vi "StartMeas.vi"(8 "error in (no error)":errorcluster, 11 "ChromaAcLoad in":refnum<class "ChromaAcLoad.lvclass">) -> (0 "error out":errorcluster, 3 "ChromaAcLoad out":refnum<class "ChromaAcLoad.lvclass">)   [LabVIEW 2018, in "AcPwrPlugins.lvlib" / "ChromaAcLoad.lvclass"]
uses:
  ChromaAcLoad.lvclass
  C:/Users/ico/Documents/Projects/NistPluggableModules/AcPwr/AcPwrPlugins/AcPwrBaseClass/AcPwrBase.lvclass
  AcPwrBaseClass/AcPwrBase.lvclass/AcPwrBase.ctl
  AcPwrBaseClass/Accessors/Read BaseMeasures.vi
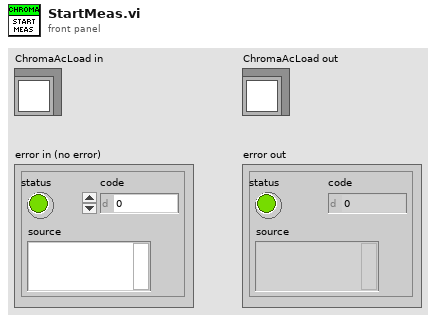
[diagram p1: front panel]
types:
  T1 = typedef "AcPwrPlugins.lvlib/AcPwrBase.lvclass/BaseMeasure.ctl" = cluster{"Handle":string, "Name":string, "Enabled":bool, "Result":dbl, "MeasType":T2, "btnMeasFetch":bool, "Hold Peak?":bool}
  T2 = typedef "AcPwrPlugins.lvlib/AcPwrBase.lvclass/MeasType.ctl" = enum16{"Voltage RMS L-N", "Current RMS", "Frequency", "Voltage DC", "Current DC", "Power Factor", "Current Peak", "Power VA", "Real Power", "Voltage THD", "Voltage EHD", "Voltage OHD", "Current THD", "Current EHD", "Current OHD", "Voltage RMS L-L", "Phase Angle", "Power DC", "Crest Factor"}
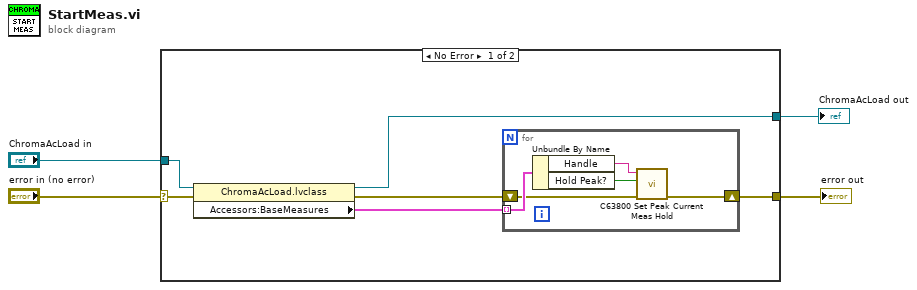
[diagram p0: block diagram]
diagram:
  n1 = case shown="No Error" "error in (no error)" {
    selector: "error in (no error)" -> [w8 w17]
    tunnel: "ChromaAcLoad in" -> [w10 w16]
    tunnel: [w9 w16] -> w3
    tunnel: [w5 w17] -> w1
    frame No Error {
      n2 = property class="ChromaAcLoad.lvclass"(reference=w10, error in=w8) -> (reference out=w9:refnum<class "ChromaAcLoad.lvclass">, error out=w6:errorcluster, "Accessors:BaseMeasures"=w7:T1[])
      n3 = for {
        tunnel: w7 -> [w15] mode=indexing
        shift-right: [w11] -> w5
        shift-left: w6 -> [w12]
        n4 = Unbundle By Name(w15) -> ("Handle"=w14:string, "Hold Peak?"=w13:bool)
        n5 = call <instrlib>:"C63800 Set Peak Current Meas Hold.vi"("error in (no error)"=w12, "Hold State"=w13, "Instrument Handle"=w14) -> ("error out"=w11:errorcluster)  [unwired: 7 in, 1 out]
      }
    }
    frame Error {
    }
  }
  "error out" <- w1
  "ChromaAcLoad out" <- w3
